vi "DSF.Engine.Memory.ObjectPool.Destroy.vi"(8 "error in (no error)":errorcluster, 11 "ObjectPool":refnum<class "DSF.Engine.Memory.ObjectPool.lvclass">) -> (0 "error out":errorcluster, 3 "Objects":refnum<class>[](array[class]))   [LabVIEW 2016, in "DSF.Engine.lvlib" / "DSF.Engine.Memory.ObjectPool.lvclass"]
uses:
  DSF.Engine.Memory.ObjectPool.lvclass
  DSF.Engine.Memory.ObjectPool.lvclass/DSF.Engine.Memory.ObjectPool.ctl
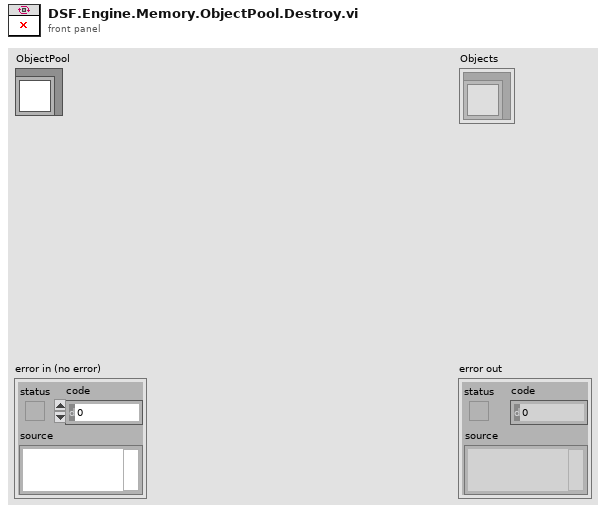
[diagram p1: front panel]
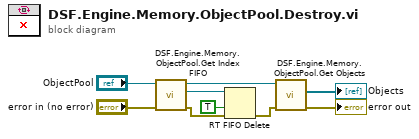
[diagram p0: block diagram]
diagram:
  n1 = call "DSF.Engine.Memory.ObjectPool.Get Index FIFO.vi"("error in (no error)"="error in (no error)", "ObjectPool in"="ObjectPool") -> ("error out"=w3:errorcluster, "Index FIFO"=w1:refnum<k33>, "ObjectPool out"=w8:refnum<class "DSF.Engine.Memory.ObjectPool.lvclass">)  [unwired: 7 in]
  n2 = RT FIFO Delete(0:w1, 2:TRUE ("force destroy? (F)"), 3:w3) -> (11:w2:errorcluster)
  n3 = call "DSF.Engine.Memory.ObjectPool.Get Objects.vi"("error in (no error)"=w2, "ObjectPool in"=w8) -> ("error out"=→"error out":errorcluster, "Objects"=→"Objects":refnum<class>[])  [unwired: 7 in, 1 out]
